vi "SOUR_POW_CORR_OFFS_MAGN.vi"(0 "VISA IN":refnum<visa-resource-name>, 1 "Port number":i32, 2 "Gain or Loss(dB)":dbl, 5 "error in":errorcluster, 7 "Channel":i32) -> (14 "VISA Out":refnum<visa-resource-name>, 19 "error out":errorcluster)   [LabVIEW 2018, in "PNA-X.lvlib"]
doc: "SOURce<cnum>:POWer<port>:CORRection:OFFSet[:MAGNitude] <num>[,src] \n(Read-Write) Sets or returns a power level offset from the PNA test port power. This can be a gain or \nloss value (in dB) to account for components you connect between the source and the reference plane \nof your measurement. For example, specify 10 dB to account for a 10 dB amplifier at the input of your \nDUT. \nCal power is the sum of the test port power setting and this offset value. Following the calibration, the \nPNA power readouts are adjusted to the cal power. \nParameters \n<cnum> Any existing channel number. If unspecified, value is set to 1 \n<port> Port number to correct for source power. If unspecified, value is set to 1. \n<num> Gain or loss value in dB. Choose a value between -200 and 200 \n[src] String. (NOT case sensitive). Source port. Optional. Use SOUR:CAT? to \nreturn a list of valid port names. \nWhile this argument can be used to make settings for ALL ports, it is designed \nto access ports that are not simple numbers, such as \"Port 1 Src2\". Otherwise, \nthe <port> argument performs the same function. If both arguments are \nspecified, [src] takes priority. \nExamples SOUR:POW:CORR:OFFS 10 \nsource1:power2:correction:offset:magnitude -3 \nQuery Syntax SOURce:POWer:CORRection:OFFSet[:MAGNitude]? [src] \nReturn Type Numeric \nDefault 0 dB"
uses:
  PNA-X.lvlib
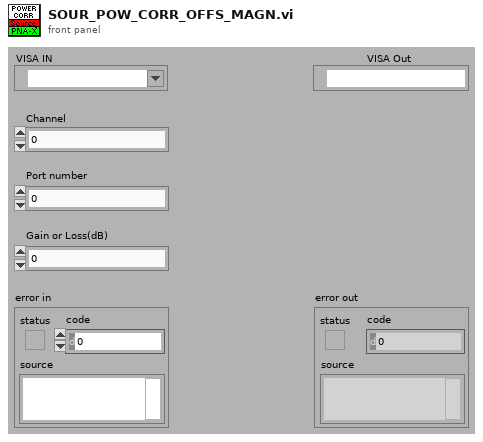
[diagram p1: front panel]
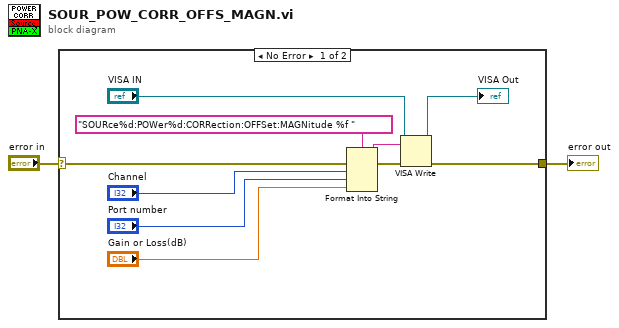
[diagram p0: block diagram]
diagram:
  n1 = case shown="No Error" "error in" {
    selector: "error in" -> [w12 w13]
    tunnel: [w7 w13] -> w1
    frame No Error {
      n2 = Format Into String(format string="SOURce%d:POWer%d:CORRection:OFFSet:MAGNitude %f " ("Cmdline"), error in=w12, "Channel", "Port number", "Gain or Loss(dB)") -> (resulting string=w10:string, error out=w11:errorcluster)  [unwired: 1 in]
      n3 = VISA Write(VISA resource name="VISA IN", write buffer=w10, error in (no error)=w11) -> (VISA resource name out=→"VISA Out":refnum<visa-resource-name>, error out=w7:errorcluster)  [unwired: 1 out]
    }
    frame Error {
    }
  }
  "error out" <- w1
